vi "FTW-Listener-Destroy.vi"(0 "FTW-Listener-TCP In":refnum<class "FTW-Listener-TCP.lvclass">, 11 "error in":errorcluster) -> (15 "error out":errorcluster)   [LabVIEW 2013, in "FTW-Listener-TCP.lvclass"]
uses:
  FTW-Listener-TCP.lvclass
  FTW-Listener-TCP.lvclass/FTW-Listener-TCP.ctl
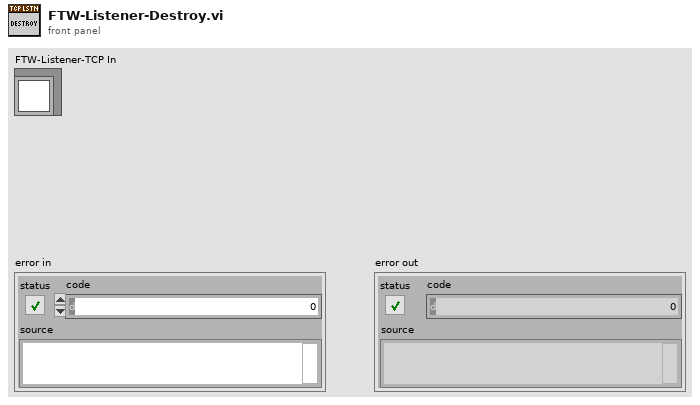
[diagram p1: front panel]
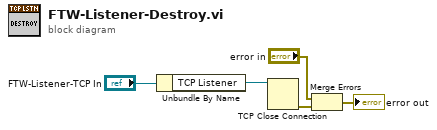
[diagram p0: block diagram]
diagram:
  n1 = Unbundle By Name("FTW-Listener-TCP In") -> ("TCP Listener"=w3:refnum<k5>)
  n2 = TCP Close Connection(connection ID=w3) -> (error out=w1:errorcluster)  [unwired: 2 in, 1 out]
  n3 = Merge Errors("error in", w1) -> (→"error out":errorcluster)
